vi "SendCommand().vi"(7 "CMD":string, 8 "error in (no error)":errorcluster, 11 "Picomoto8742ControllerClass in":refnum<class "Picomoto8742ControllerClass.lvclass">) -> (0 "error out":errorcluster, 3 "Picomoto8742ControllerClass Out":refnum<class "Picomoto8742ControllerClass.lvclass">)   [LabVIEW 2013, in "Picomoto8742ControllerClass.lvclass"]
doc: "Send a generic command to the physical device"
uses:
  Picomoto8742ControllerClass.lvclass
  Picomoto8742ControllerClass.lvclass/Picomoto8742ControllerClass.ctl
  PicoMotor8742Comm.lvclass
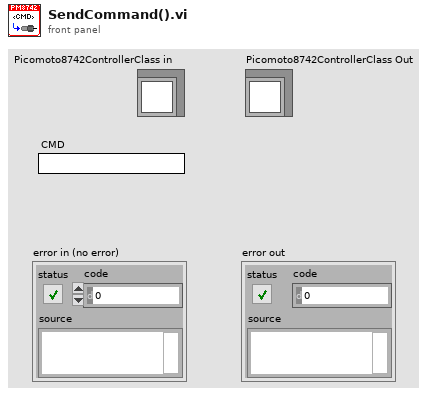
[diagram p1: front panel]
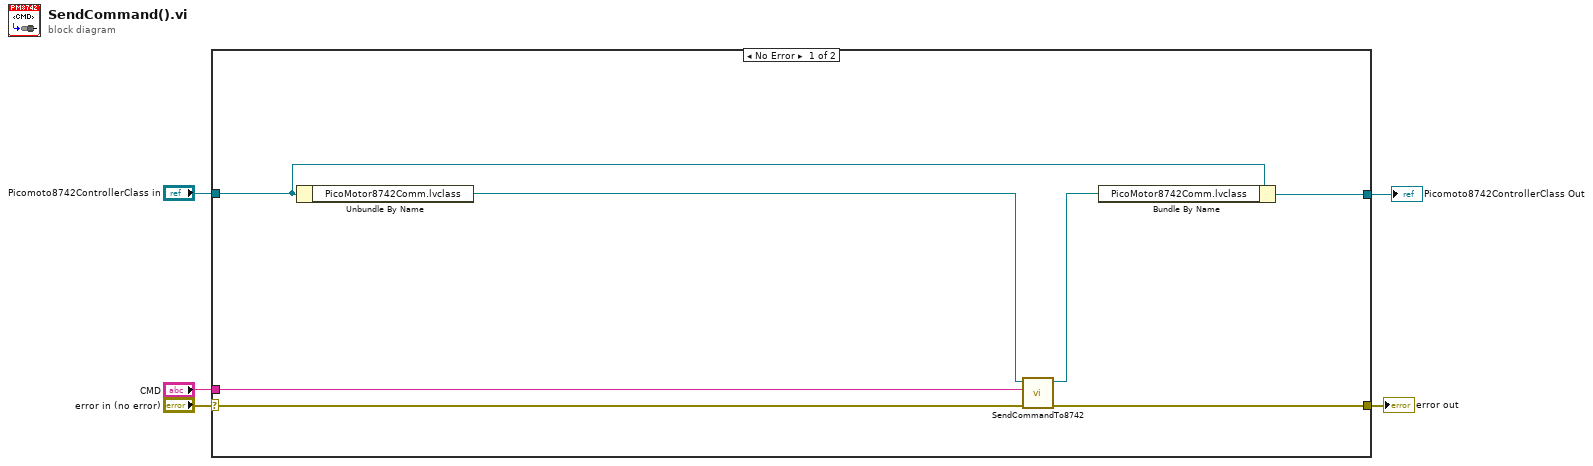
[diagram p0: block diagram]
diagram:
  n1 = case shown="No Error" "error in (no error)" {
    selector: "error in (no error)" -> [w12 w14]
    tunnel: [w11 w14] -> w5
    tunnel: "Picomoto8742ControllerClass in" -> [w8 w13]
    tunnel: [w9 w13] -> w2
    tunnel: "CMD" -> [w6 _]
    frame No Error {
      n2 = Unbundle By Name(w8) -> ("PicoMotor8742Comm.lvclass"=w7:refnum<class "PicoMotor8742Comm.lvclass">)
      n3 = call-dynamic "SendCommandTo8742.vi"("error in (no error)"=w12, "Command"=w6, "PicoMotor8742Comm in"=w7) -> ("error out"=w11:errorcluster, "PicoMotor8742Comm out"=w10:refnum<class "PicoMotor8742Comm.lvclass">)  [unwired: 6 in, 1 out]
      n4 = Bundle By Name(cluster=w8, "PicoMotor8742Comm.lvclass"=w10) -> (w9:refnum<class "Picomoto8742ControllerClass.lvclass">)
    }
    frame Error {
    }
  }
  "error out" <- w5
  "Picomoto8742ControllerClass Out" <- w2
